vi "Readout_Spectrum.vi"(0 "tdms file in":refnum<k34>, 5 "Ch_in":T1, 12 "group name":string, 13 "channel names":string[](array[string])) -> (4 "tdms file out":refnum<k34>, 6 "Ch_out":cluster{dbl[], dbl[], dbl[], dbl[]}, 14 "Spectrum_out":T2(array[cluster]))   [LabVIEW 2019]
uses:
  SiPM_Tests_Global_Var.vi
  Agilent_lib/Public/Data/Read Measurement (Current Value).vi
  Agilent_lib/Agilent 2000 3000 X-Series.lvlib
  <vilib>/Analysis/NI_AALPro.lvlib
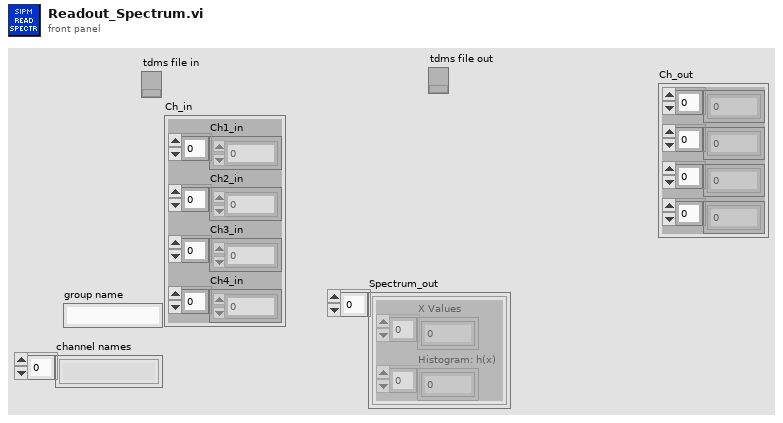
[diagram p1: front panel]
types:
  T1 = cluster{"Ch1_in":dbl[], "Ch2_in":dbl[], "Ch3_in":dbl[], "Ch4_in":dbl[]}
  T2 = cluster{"X Values":dbl[], "Histogram: h(x)":i32[]}[]
  T3 = cluster{"X Values":dbl[], "Histogram: h(x)":i32[]}
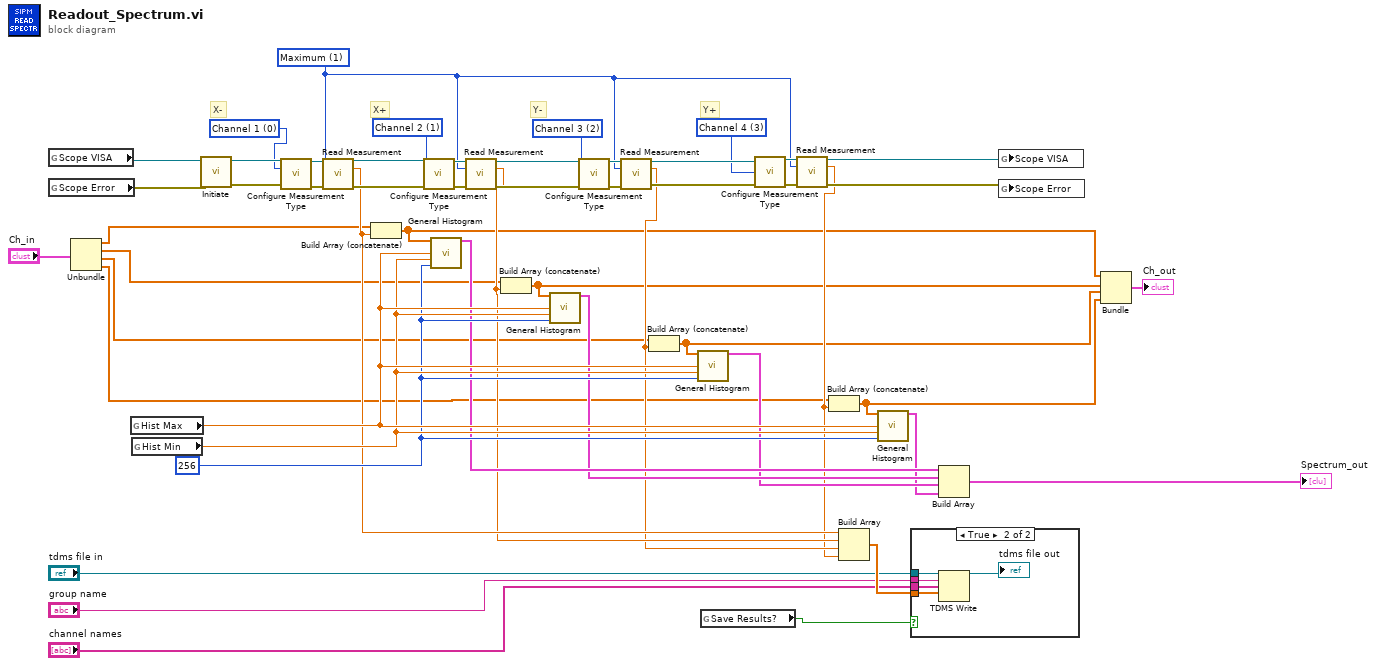
[diagram p0: block diagram]
diagram:
  w2 = 1 items=["Peak-Peak", "Maximum", "Mimimum", "Amplitude", "Top", "Base", "Overshoot", "Preshoot", "Average - N Cycles", "Average - Full Screen", "DC RMS - N Cycles", "DC RMS - Full Screen", "AC RMS - N Cycles", "AC RMS - Full Screen (Std Dev)", "Ratio", "Period", "Frequency", "Counter", "+Width", "-Width", "Burst Width", "Duty Cycle", "Rise Time", "Fall Time", "Delay", "Phase", "X minY", "X maxY", "Positive Pulse Count", "Negative Pulse Count", "Raising Edge Count", "Falling Edge Count", "Area - N Cycle", "Area - Full Screen", "Nth Edge Time", "Nth Edge Cross Level Time"] ("Measurement Type (0: Peak-Peak)")
  w32 = 0 items=["Channel 1"=0, "Channel 2"=1, "Channel 3"=2, "Channel 4"=3, "Math"=4, "Waveform Memory 1"=5, "Waveform Memory 2"=6, "D0"=13, "D1"=14, "D2"=15, "D3"=16, "D4"=17, "D5"=18, "D6"=19, "D7"=20, "D8"=21, "D9"=22, "D10"=23, "D11"=24, "D12"=25, "D13"=26, "D14"=27, "D15"=28, "External"=29, "Function"=32] ("Measurement Source 1 (0: Channel 1)")
  w33 = 3 items=["Channel 1"=0, "Channel 2"=1, "Channel 3"=2, "Channel 4"=3, "Math"=4, "Waveform Memory 1"=5, "Waveform Memory 2"=6, "D0"=13, "D1"=14, "D2"=15, "D3"=16, "D4"=17, "D5"=18, "D6"=19, "D7"=20, "D8"=21, "D9"=22, "D10"=23, "D11"=24, "D12"=25, "D13"=26, "D14"=27, "D15"=28, "External"=29, "Function"=32] ("Measurement Source 1 (0: Channel 1)")
  w29 = 256 ("# bins")
  w48 = 2 items=["Channel 1"=0, "Channel 2"=1, "Channel 3"=2, "Channel 4"=3, "Math"=4, "Waveform Memory 1"=5, "Waveform Memory 2"=6, "D0"=13, "D1"=14, "D2"=15, "D3"=16, "D4"=17, "D5"=18, "D6"=19, "D7"=20, "D8"=21, "D9"=22, "D10"=23, "D11"=24, "D12"=25, "D13"=26, "D14"=27, "D15"=28, "External"=29, "Function"=32] ("Measurement Source 1 (0: Channel 1)")
  w43 = 1 items=["Channel 1"=0, "Channel 2"=1, "Channel 3"=2, "Channel 4"=3, "Math"=4, "Waveform Memory 1"=5, "Waveform Memory 2"=6, "D0"=13, "D1"=14, "D2"=15, "D3"=16, "D4"=17, "D5"=18, "D6"=19, "D7"=20, "D8"=21, "D9"=22, "D10"=23, "D11"=24, "D12"=25, "D13"=26, "D14"=27, "D15"=28, "External"=29, "Function"=32] ("Measurement Source 1 (0: Channel 1)")
  # "Y-"
  # "Y+"
  # "X-"
  # "X+"
  n1 = global read "SiPM_Tests_Global_Var.vi" "Scope VISA"() -> (w49:refnum<visa-resource-name>)
  n2 = global read "SiPM_Tests_Global_Var.vi" "Scope Error"() -> (w50:errorcluster)
  n3 = Unbundle("Ch_in") -> ("Ch1_in"=w12:dbl[], "Ch2_in"=w11:dbl[], "Ch3_in"=w10:dbl[], "Ch4_in"=w9:dbl[])
  n4 = global read "SiPM_Tests_Global_Var.vi" "Hist Max"() -> (w31:dbl)
  n5 = global read "SiPM_Tests_Global_Var.vi" "Hist Min"() -> (w30:dbl)
  n6 = call "Initiate.vi"("error in (no error)"=w50, "VISA resource name"=w49) -> ("error out"=w51:errorcluster, "VISA resource name out"=w52:refnum<visa-resource-name>)  [unwired: 8 in]
  n7 = call "Configure Measurement Type.vi"("VISA resource name"=w52, "Measurement Type (0: Peak-Peak)"=w32, "error in (no error)"=w51) -> ("VISA resource name out"=w37:refnum<visa-resource-name>, "error out"=w38:errorcluster)  [unwired: 11 in]
  n8 = call-poly "Read Measurement.vi"("VISA resource name"=w37, "Measurement Type (0: Peak-Peak)"=w2, "error in (no error)"=w38) -> ("VISA resource name out"=w40:refnum<visa-resource-name>, "Result Value"=w18:dbl, "error out"=w41:errorcluster)  [unwired: 10 in]
  n9 = Build Array (concatenate)(w12, w18) -> (w8:dbl[])
  n10 = call "Configure Measurement Type.vi"("VISA resource name"=w40, "Measurement Source 1 (0: Channel 1)"=w43, "error in (no error)"=w41) -> ("VISA resource name out"=w42:refnum<visa-resource-name>, "error out"=w39:errorcluster)  [unwired: 11 in]
  n11 = call <vilib>:"General Histogram.vi"("X"=w8, "max"=w31, "min"=w30, "# bins"=w29) -> ("Histogram Graph"=w28:T3)  [unwired: 7 in, 4 out]
  n12 = call-poly "Read Measurement.vi"("VISA resource name"=w42, "Measurement Type (0: Peak-Peak)"=w2, "error in (no error)"=w39) -> ("VISA resource name out"=w44:refnum<visa-resource-name>, "Result Value"=w17:dbl, "error out"=w45:errorcluster)  [unwired: 10 in]
  n13 = Build Array (concatenate)(w11, w17) -> (w7:dbl[])
  n14 = call <vilib>:"General Histogram.vi"("X"=w7, "max"=w31, "min"=w30, "# bins"=w29) -> ("Histogram Graph"=w27:T3)  [unwired: 7 in, 4 out]
  n15 = call "Configure Measurement Type.vi"("VISA resource name"=w44, "Measurement Source 1 (0: Channel 1)"=w48, "error in (no error)"=w45) -> ("VISA resource name out"=w46:refnum<visa-resource-name>, "error out"=w47:errorcluster)  [unwired: 11 in]
  n16 = call-poly "Read Measurement.vi"("VISA resource name"=w46, "Measurement Type (0: Peak-Peak)"=w2, "error in (no error)"=w47) -> ("VISA resource name out"=w35:refnum<visa-resource-name>, "Result Value"=w16:dbl, "error out"=w34:errorcluster)  [unwired: 10 in]
  n17 = Build Array (concatenate)(w10, w16) -> (w6:dbl[])
  n18 = call <vilib>:"General Histogram.vi"("X"=w6, "max"=w31, "min"=w30, "# bins"=w29) -> ("Histogram Graph"=w26:T3)  [unwired: 7 in, 4 out]
  n19 = global read "SiPM_Tests_Global_Var.vi" "Save Results?"() -> (w14:bool)
  n20 = call "Configure Measurement Type.vi"("VISA resource name"=w35, "Measurement Source 1 (0: Channel 1)"=w33, "error in (no error)"=w34) -> ("VISA resource name out"=w36:refnum<visa-resource-name>, "error out"=w3:errorcluster)  [unwired: 11 in]
  n21 = call-poly "Read Measurement.vi"("VISA resource name"=w36, "Measurement Type (0: Peak-Peak)"=w2, "error in (no error)"=w3) -> ("VISA resource name out"=w24:refnum<visa-resource-name>, "Result Value"=w15:dbl, "error out"=w23:errorcluster)  [unwired: 10 in]
  n22 = Build Array (concatenate)(w9, w15) -> (w5:dbl[])
  n23 = Build Array(w18, w17, w16, w15) -> (w22:dbl[])
  n24 = call <vilib>:"General Histogram.vi"("X"=w5, "max"=w31, "min"=w30, "# bins"=w29) -> ("Histogram Graph"=w25:T3)  [unwired: 7 in, 4 out]
  n25 = case shown="True" w14 {
    tunnel: w22 -> [_ w57]
    tunnel: "tdms file in" -> [_ w55]
    tunnel: "group name" -> [_ w54]
    tunnel: "channel names" -> [_ w53]
    frame False {
    }
    frame True {
      n26 = TDMS Write(0:w55, 5:w54, 7:w53, 9:w57) -> (4:→"tdms file out":refnum<k34>)  [unwired: 2 in, 3 out]
    }
  }
  n27 = Build Array(w28, w27, w26, w25) -> (→"Spectrum_out":T2)
  n28 = global write "SiPM_Tests_Global_Var.vi" "Scope VISA"(w24) -> ()
  n29 = global write "SiPM_Tests_Global_Var.vi" "Scope Error"(w23) -> ()
  n30 = Bundle(w8, w7, w6, w5) -> (→"Ch_out":cluster{dbl[], dbl[], dbl[], dbl[]})  [unwired: 1 in]
